vi "dg535 delay.vi"(1 "C":dbl min=0.0 max=999.999999999995 format="%.12f", 2 "D":dbl min=0.0 max=999.999999999995 format="%.12f", 3 "D=":u32(slide) scale=0.0..3.0, 4 "C=":u32(slide) scale=0.0..3.0, 5 "B":dbl min=0.0 max=999.999999999995 format="%.12f", 6 "error in":errorcluster, 7 "A":dbl min=0.0 max=999.999999999995 format="%.12f", 8 "B=":u32(slide) scale=0.0..3.0, 9 "A=":u32(slide) scale=0.0..3.0, 10 "GPIB address":string="15") -> (0 "error out":errorcluster)   [LabVIEW 2013]
doc: "This subVI sets the delay of the output channels relative to other channels or to the time reference T0 .\nControls A=, B= , C= and D= specify the reference channel and \nA, B, C, and D set the delay time in seconds .\nA Delay Linkage Error will be caused by an attempt to totally disconnect a time reference from T0 ."
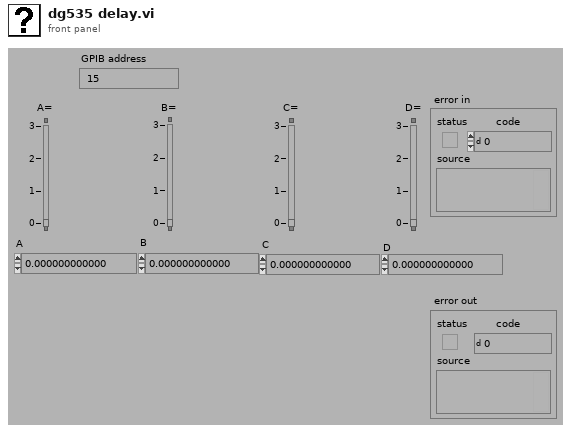
[diagram p1: front panel]
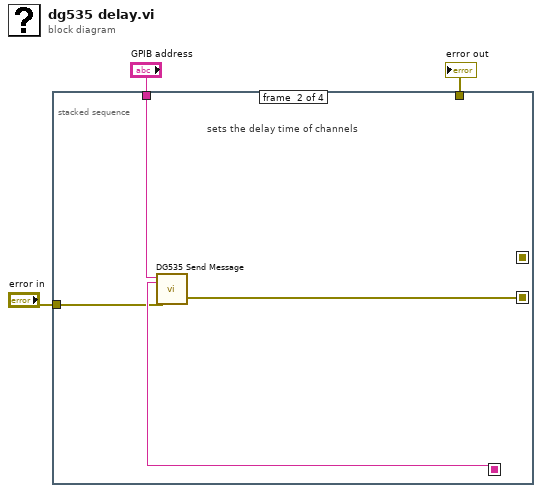
[diagram p0: block diagram]
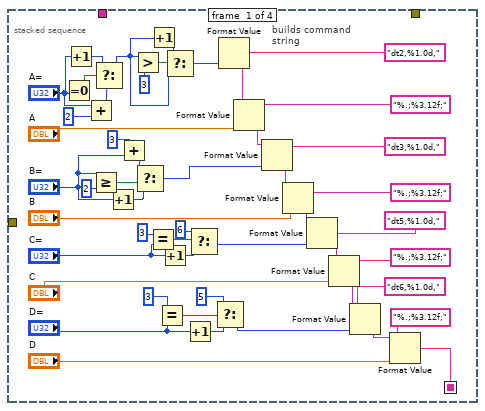
[diagram p2: hidden frame]
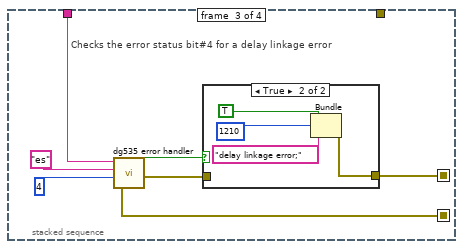
[diagram p3: hidden frame]
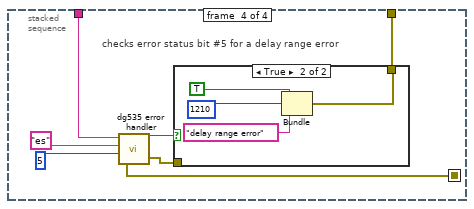
[diagram p5: hidden frame]
diagram:
  n1 = stacked-sequence {
    seq-local: [w34 _ _ _] -> [_ w55 _ _]
    seq-local: [_ w53 _ _] -> [_ _ w62 _]
    seq-local: [_ _ w59 _] -> [_ _ _ w69]
    tunnel: "GPIB address" -> [_ w56 w63 w72]
    tunnel: "error in" -> [_ w54 _ _]
    tunnel: [_ _ _ w73] -> w2
    frame #0 {
      # "builds command\nstring"
      n2 = Equal To 0?(x="A=") -> (x = 0?=w15:bool)
      n3 = Increment(x="A=") -> (x+1=w5:u32)
      n4 = Add(x="A=", y=2) -> (x+y=w12:u32)
      n5 = Greater Or Equal?(x="B=", y=2) -> (x >= y?=w18:bool)
      n6 = Select(t=w5, s=w15, f=w12) -> (s? t:f=w4:u32)
      n7 = Increment(x="B=") -> (x+1=w16:u32)
      n8 = Add(x=3, y="B=") -> (x+y=w19:u32)
      n9 = Greater?(x=w4, y=3) -> (0:w10:bool)
      n10 = Select(t=w19, s=w18, f=w16) -> (s? t:f=w17:u32)
      n11 = Equal?(x=3, y="C=") -> (x = y?=w26:bool)
      n12 = Increment(x=w4) -> (x+1=w9:u32)
      n13 = Equal?(x=3, y="D=") -> (x = y?=w31:bool)
      n14 = Increment(x="C=") -> (x+1=w22:u32)
      n15 = Select(t=w9, s=w10, f=w4) -> (s? t:f=w8:u32)
      n16 = Increment(x="D=") -> (x+1=w24:u32)
      n17 = Select(t=6, s=w26, f=w22) -> (s? t:f=w21:u32)
      n18 = Select(t=5, s=w31, f=w24) -> (s? t:f=w28:u32)
      n19 = Format Value(format string="dt2,%1.0d,", value (0)=w8) -> (output string=w45:string)  [unwired: 1 in]
      n20 = Format Value(string ("")=w45, format string="%.;%3.12f;", value (0)="A") -> (output string=w44:string)
      n21 = Format Value(string ("")=w44, format string="dt3,%1.0d,", value (0)=w17) -> (output string=w48:string)
      n22 = Format Value(string ("")=w48, format string="%.;%3.12f;", value (0)="B") -> (output string=w33:string)
      n23 = Format Value(string ("")=w33, format string="dt5,%1.0d,", value (0)=w21) -> (output string=w37:string)
      n24 = Format Value(string ("")=w37, format string="%.;%3.12f;", value (0)="C") -> (output string=w35:string)
      n25 = Format Value(string ("")=w35, format string="dt6,%1.0d,", value (0)=w28) -> (output string=w42:string)
      n26 = Format Value(string ("")=w42, format string="%.;%3.12f;", value (0)="D") -> (output string=w34:string)
    }
    frame #1 {
      # "sets the delay time of channels"
      n27 = call "DG535 Send Message.vi"("address string"=w56, "write buffer"=w55, "error in"=w54) -> ("error out"=w53:errorcluster)  [unwired: 4 in, 2 out]
    }
    frame #2 {
      # "Checks the error status bit#4 for a delay linkage error"
      n28 = call "dg535 error handler.vi"("error in"=w62, "check bit #"=4, "command string"="es", "GPIB address"=w63) -> ("error out"=w60:errorcluster, "error found"=w61:bool)
      n29 = case shown="True" w61 {
        tunnel: w60 -> [w64 _]
        tunnel: [w64 w65] -> w59
        frame False {
        }
        frame True {
          n30 = Bundle(TRUE, 1210, "delay linkage error;") -> (w65:errorcluster)  [unwired: 1 in]
        }
      }
    }
    frame #3 {
      # "checks error status bit #5 for a delay range error"
      n31 = call "dg535 error handler.vi"("error in"=w69, "check bit #"=5, "command string"="es", "GPIB address"=w72) -> ("error out"=w74:errorcluster, "error found"=w75:bool)
      n32 = case shown="True" w75 {
        tunnel: w74 -> [w76 _]
        tunnel: [w76 w77] -> w73
        frame False {
        }
        frame True {
          n33 = Bundle(TRUE, 1210, "delay range error") -> (w77:errorcluster)  [unwired: 1 in]
        }
      }
    }
  }
  "error out" <- w2
